vi "Periodic Tasks.vi"(8 "error in (no error)":errorcluster) -> ()   [LabVIEW 2014]
doc: "This VI runs in parallel to other tasks. It can contain as many user-defined periodic loops as you need. These can carry out PID or other sorts of timed response."
uses:
  Robot Global Data.vi
  <vilib>/Rock Robotics/WPI/Solenoid/Deprecated/WPI_SolenoidSetBool.vi
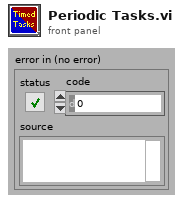
[diagram p1: front panel]
types:
  T1 = typedef "WPI_SolenoidDevRef.ctl" = cluster{"DevStatus":errorcluster, "Pneumatics Control Module":u8, "Forward Solenoid Channel":T2, "Reverse Solenoid Channel":T2}
  T2 = typedef "WPI_SolenoidChannel.ctl" = enum8{"Solenoid 0", "Solenoid 1", "Solenoid 2", "Solenoid 3", "Solenoid 4", "Solenoid 5", "Solenoid 6", "Solenoid 7", "Invalid"}
  T3 = typedef "WPI_CameraDevRef.ctl" = cluster{"Camera Address":string, "CameraStatus":errorcluster}
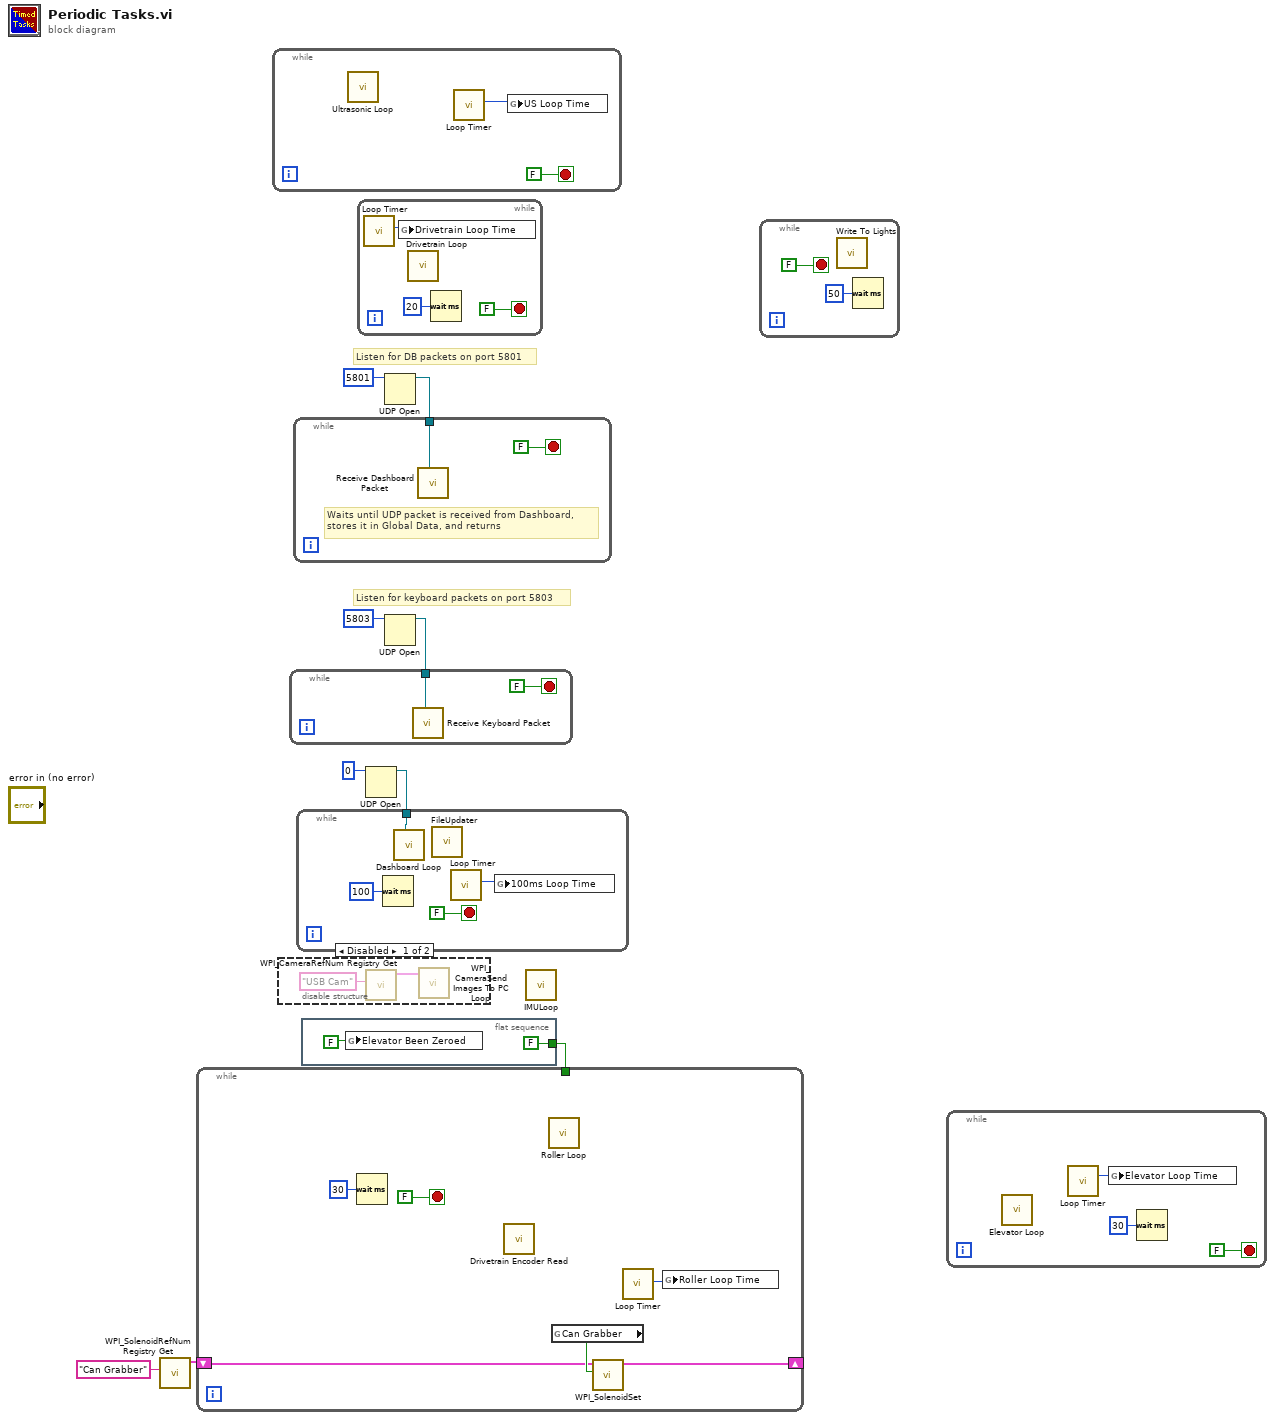
[diagram p0: block diagram]
diagram:
  # "Listen for keyboard packets on port 5803"
  # "Listen for DB packets on port 5801"
  n1 = call <vilib>:"WPI_SolenoidRefNum Registry Get.vi"("refnum name"="Can Grabber") -> ("SolenoidDevRef"=w1:T1)  [unwired: 9 in, 1 out]
  n2 = while {
    tunnel: w2 -> [_]
    shift-right: [w11] -> _
    shift-left: w1 -> [w10]
    stop <- FALSE stop-if-true
    n3 = Wait (ms)(milliseconds to wait=u32 30) -> ()  [unwired: 1 out]
    n4 = call "Drivetrain Encoder Read.vi"() -> ()  [unwired: 11 in, 1 out]
    n5 = call "Roller Loop.vi"() -> ()  [unwired: 12 in]
    n6 = global read "Robot Global Data.vi" "Can Grabber"() -> (w12:bool)
    n7 = call-poly <vilib>:"WPI_SolenoidSet.vi"("Value"=w12, "SolenoidDevRef"=w10) -> ("SolenoidDevRef"=w11:T1)  [unwired: 8 in, 1 out]
    n8 = call "Loop Timer.vi"() -> ("dt"=w13:u32)  [unwired: 11 in]
    n9 = global write "Robot Global Data.vi" "Roller Loop Time"(w13) -> ()
  }
  n10 = while {
    stop <- FALSE stop-if-true
    n11 = call "Ultrasonic Loop.vi"() -> ()  [unwired: 12 in]
    n12 = call "Loop Timer.vi"() -> ("dt"=w16:u32)  [unwired: 11 in]
    n13 = global write "Robot Global Data.vi" "US Loop Time"(w16) -> ()
  }
  n14 = disable-structure shown="Disabled" {
    frame Disabled {
      n15 = call <vilib>:"WPI_CameraRefNum Registry Get.vi"("refnum name"="USB Cam") -> ("CameraDevRef"=w19:T3)  [unwired: 9 in, 1 out]
      n16 = call <vilib>:"WPI_CameraSend Images To PC Loop.vi"("CameraDevRef"=w19) -> ()  [unwired: 11 in]
    }
    frame Enabled {
    }
  }
  n17 = flat-sequence {
    tunnel: [FALSE] -> w2
    frame #0 {
      n18 = global write "Robot Global Data.vi" "Elevator Been Zeroed"(FALSE) -> ()
    }
  }
  n19 = while {
    stop <- FALSE stop-if-true
    n20 = call "Loop Timer.vi"() -> ("dt"=w22:u32)  [unwired: 11 in]
    n21 = global write "Robot Global Data.vi" "Drivetrain Loop Time"(w22) -> ()
    n22 = call "Drivetrain Loop.vi"() -> ()  [unwired: 12 in]
    n23 = Wait (ms)(milliseconds to wait=u32 20) -> ()  [unwired: 1 out]
  }
  n24 = UDP Open(11:u16 0 ("port")) -> (port=w7:refnum<k16>)  [unwired: 4 in, 2 out]
  n25 = while {
    tunnel: w7 -> [w26]
    stop <- FALSE stop-if-true
    n26 = Wait (ms)(milliseconds to wait=u32 100) -> ()  [unwired: 1 out]
    n27 = call "Dashboard Loop.vi"("connection ID"=w26) -> ()  [unwired: 11 in]
    n28 = call "FileUpdater.vi"() -> ()  [unwired: 12 in]
    n29 = call "Loop Timer.vi"() -> ("dt"=w25:u32)  [unwired: 11 in]
    n30 = global write "Robot Global Data.vi" "100ms Loop Time"(w25) -> ()
  }
  n31 = UDP Open(11:u16 5801 ("port")) -> (port=w9:refnum<k16>)  [unwired: 4 in, 2 out]
  n32 = while {
    tunnel: w9 -> [w29]
    stop <- FALSE stop-if-true
    # "Waits until UDP packet is received from Dashboard,\nstores it in Global Data, and returns"
    n33 = call "Receive Dashboard Packet.vi"("connection ID"=w29) -> ()  [unwired: 11 in]
  }
  n34 = UDP Open(11:u16 5803 ("port")) -> (port=w4:refnum<k16>)  [unwired: 4 in, 2 out]
  n35 = while {
    tunnel: w4 -> [w31]
    stop <- FALSE stop-if-true
    n36 = call "Receive Keyboard Packet.vi"("connection ID"=w31) -> ()  [unwired: 11 in]
  }
  n37 = call "IMULoop.vi"() -> ()  [unwired: 12 in]
  n38 = while {
    stop <- FALSE stop-if-true
    n39 = call "Write To Lights.vi"() -> ()  [unwired: 12 in]
    n40 = Wait (ms)(milliseconds to wait=u32 50) -> ()  [unwired: 1 out]
  }
  n41 = while {
    stop <- FALSE stop-if-true
    n42 = call "Elevator Loop.vi"() -> ()  [unwired: 12 in]
    n43 = call "Loop Timer.vi"() -> ("dt"=w37:u32)  [unwired: 11 in]
    n44 = global write "Robot Global Data.vi" "Elevator Loop Time"(w37) -> ()
    n45 = Wait (ms)(milliseconds to wait=u32 30) -> ()  [unwired: 1 out]
  }
